vi "Close.vi"(8 "error in":errorcluster, 11 "Error Channels in":refnum<class "Error Channels.lvclass">) -> (0 "error out":errorcluster, 3 "Error Channels out":refnum<class "Error Channels.lvclass">)   [LabVIEW 2023, in "Error Channels.lvclass"]
uses:
  Error Channels.lvclass
  Error Channels.lvclass/Error Channels.ctl
  <vilib>/ADAS Replay HIL/AdasHilServices/AdasHilChannelServices.lvlib
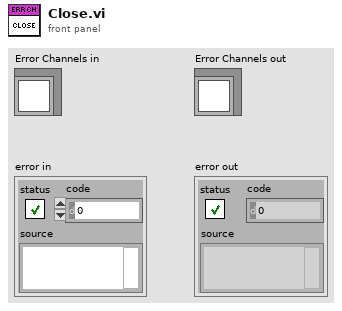
[diagram p1: front panel]
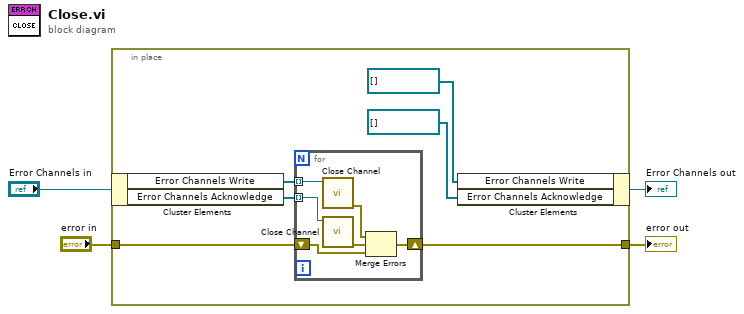
[diagram p0: block diagram]
diagram:
  n1 = in-place {
    in-place-border: [w10] -> w1
    in-place-border: "error in" -> [w7]
    n2 = in-place-cluster #1("Error Channels in") -> ("Error Channels Write"=w9:refnum<k21>[], "Error Channels Acknowledge"=w6:refnum<k21>[])
    n3 = for {
      tunnel: w9 -> [w16] mode=indexing
      shift-right: [w14] -> w10
      shift-left: w7 -> [w11]
      tunnel: w6 -> [w13] mode=indexing
      n4 = call <vilib>:"Close Channel.vi"("ADAS HIL Channel"=w16) -> ("error out"=w15:errorcluster)  [unwired: 10 in]
      n5 = call <vilib>:"Close Channel.vi"("ADAS HIL Channel"=w13) -> ("error out"=w12:errorcluster)  [unwired: 10 in]
      n6 = Merge Errors(w15, w12, w11) -> (w14:errorcluster)
    }
    n7 = in-place-cluster #1("Error Channels Write"=refnum<k21>[] [] ("Actual Value Object"), "Error Channels Acknowledge"=refnum<k21>[] []) -> (→"Error Channels out":refnum<class "Error Channels.lvclass">)
  }
  "error out" <- w1
